vi "setSize.vi"(0 "HGF_Rendezvous":refnum<class "HGF_Rendezvous.lvclass">, 2 "size (2)":i32, 5 "error in (no error)":errorcluster) -> (14 "dup HGF_Rendezvous":refnum<class "HGF_Rendezvous.lvclass">, 16 "new size":i32, 19 "error out":errorcluster)   [LabVIEW 2014, in "HGF_BaseClasses.lvlib" / "HGF_Rendezvous.lvclass"]
doc: "Set size of rendezvous."
uses:
  HGF_Rendezvous.lvclass
  HGF_Auxiliary/HGF_Auxiliary.lvlib
  HGF_Auxiliary/Severity.ctl
  HGF_Auxiliary/ErrorCode.ctl
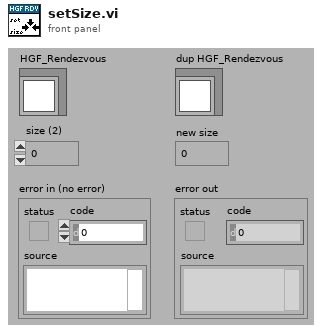
[diagram p1: front panel]
types:
  T1 = typedef "HGF_Auxiliary.lvlib/ErrorCode.ctl" = enum32{"No error", "Function not supported.", "This VI is for friends only.", "Reference object aready exisits.", "Parameter out of range.", "Not a rendezvous.", "Invalid notifier reference.", "Invalid queue reference.", "Self-Test not supported.", "Reset not supported.", "IDN query not supported.", "Error query not supported.", "Incorrect addressee.", "Object already exists.", "No class name specified", "Driver not supported", "Attribute is not writable"}
  T2 = typedef "HGF_Auxiliary.lvlib/Severity.ctl" = enum16{"Info", "Warning", "Fault", "Error", "Fatal"}
  T3 = typedef "Rendezvous RefNum" = refnum<k1>
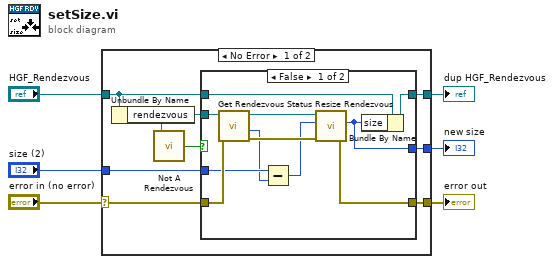
[diagram p0: block diagram]
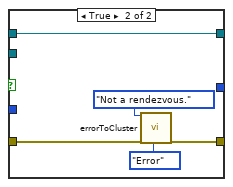
[diagram p2: hidden frame]
diagram:
  n1 = case shown="No Error" "error in (no error)" {
    selector: "error in (no error)" -> [w12 w32]
    tunnel: [w13 w32] -> w5
    tunnel: [w9 w31] -> w3
    tunnel: "HGF_Rendezvous" -> [w8 w31]
    tunnel: "size (2)" -> [w10 _]
    tunnel: [w7 _] -> w1
    frame No Error {
      n2 = Unbundle By Name(w8) -> ("rendezvous"=w11:T3)
      n3 = call <vilib>:"Not A Rendezvous.vi"("rendezvous"=w11) -> ("not a rendezvous"=w14:bool)
      n4 = case shown="False" w14 {
        tunnel: [w23 w28] -> w13
        tunnel: w12 -> [w19 w29]
        tunnel: w11 -> [w21 _]
        tunnel: w10 -> [w17 _]
        tunnel: [w24 w30] -> w9
        tunnel: w8 -> [w25 w30]
        tunnel: [w22 _] -> w7
        frame False {
          n5 = call <vilib>:"Get Rendezvous Status.vi"("error in (no error)"=w19, "rendezvous"=w21) -> ("error out"=w18:errorcluster, "size"=w16:i32, "rendezvous out"=w20:T3)  [unwired: 7 out]
          n6 = Subtract(x=w17, y=w16) -> (x-y=w15:i32)
          n7 = call <vilib>:"Resize Rendezvous.vi"("error in (no error)"=w18, "size change (0)"=w15, "rendezvous"=w20) -> ("error out"=w23:errorcluster, "new size"=w22:i32)  [unwired: 3 out]
          n8 = Bundle By Name(cluster=w25, "size"=w22) -> (w24:refnum<class "HGF_Rendezvous.lvclass">)
        }
        frame True {
          n9 = call "errorToCluster.vi"("error code"=ErrorCode."Not a rendezvous.", "error in (no error)"=w29, "severity (Error)"=Severity."Error") -> ("error out"=w28:errorcluster)  [unwired: 2 in, 14 out]
        }
      }
    }
    frame Error {
    }
  }
  "error out" <- w5
  "dup HGF_Rendezvous" <- w3
  "new size" <- w1
